vi "Advanced Cut - Auto Equal Cut.vi"(8 "error in (no error)":errorcluster, 11 "Auto Cut (Equal)":T1={"Start Time (s)"=0.0, "End Time (s)"=90.0, "# Epochs"=10} {"End Time (s)" min=0.0 step=1.0; "Start Time (s)" min=0.0 step=1.0}) -> (0 "error out":errorcluster, 3 "Snippets":dbl[][](array[numeric]))   [LabVIEW 2016]
uses:
  Type Definitions/Advanced Cut - Equal Auto Cut.ctl
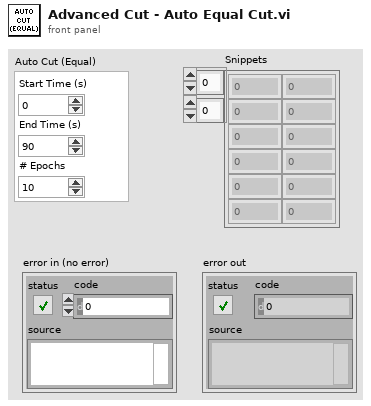
[diagram p1: front panel]
types:
  T1 = typedef "Advanced Cut - Equal Auto Cut.ctl" = cluster{"Start Time (s)":dbl, "End Time (s)":dbl, "# Epochs":u32}
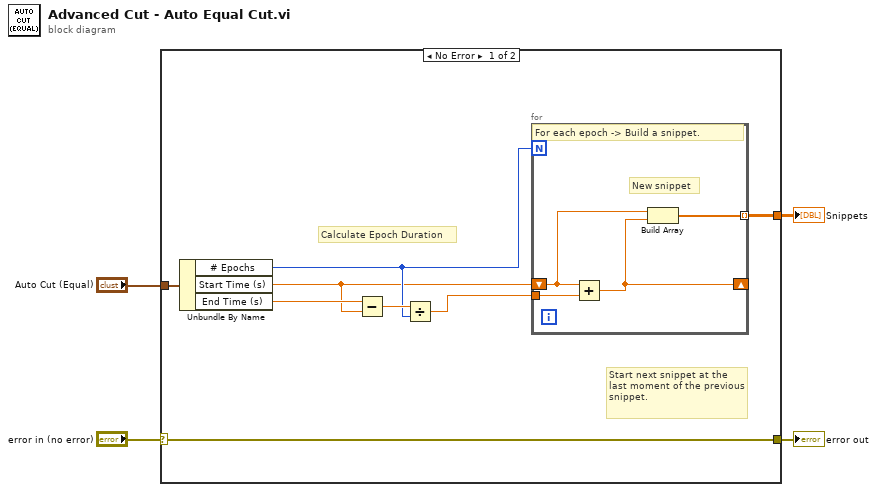
[diagram p0: block diagram]
diagram:
  n1 = case shown="No Error" "error in (no error)" {
    selector: "error in (no error)" -> [w12 w17]
    tunnel: [w12 w17] -> w3
    tunnel: [w11 _] -> w2
    tunnel: "Auto Cut (Equal)" -> [w10 _]
    frame No Error {
      # "Calculate Epoch Duration"
      # "Start next snippet at the last moment of the previous snippet."
      n2 = Unbundle By Name(w10) -> ("# Epochs"=w8:u32, "Start Time (s)"=w5:dbl, "End Time (s)"=w6:dbl)
      n3 = Subtract(x=w6, y=w5) -> (x-y=w9:dbl)
      n4 = Divide(x=w9, y=w8) -> (x/y=w7:dbl)
      n5 = for {
        N: w8 -> [_]
        shift-right: [w15] -> _
        shift-left: w5 -> [w16]
        tunnel: [w14] -> w11 mode=indexing
        tunnel: w7 -> [w13]
        # "New snippet"
        # "For each epoch -> Build a snippet."
        n6 = Add(x=w16, y=w13) -> (x+y=w15:dbl)
        n7 = Build Array(w16, w15) -> (w14:dbl[])
      }
    }
    frame Error {
    }
  }
  "error out" <- w3
  "Snippets" <- w2
